vi "angle-statstics-test.vi"(8 "error in (no error)":errorcluster) -> (0 "error out":errorcluster, 3 "All Passed":bool)   [LabVIEW 2019]
uses:
  <vilib>/Analysis/Matrix/Datatypes/RealMatrix.ctl
  <vilib>/Rock Robotics/WPI/ThirdParty/JAS_Junk/TrajLib/MatBuilder_Create.vi
  <vilib>/Rock Robotics/WPI/ThirdParty/JAS_Junk/TrajLib/MathUtil_AngleModulus.vi
  <vilib>/Rock Robotics/WPI/ThirdParty/JAS_Junk/TrajLib/Matrix_ExtractRowVector.vi
  <vilib>/Analysis/baseanly.llb/A x B.vi
  <vilib>/Analysis/baseanly.llb/Real A x B.vi
  <vilib>/Rock Robotics/WPI/ThirdParty/JAS_Junk/TrajLib/Matrix_ElementSum.vi
  <vilib>/Rock Robotics/WPI/ThirdParty/JAS_Junk/TrajLib/MathUtil_InputModulus.vi
  <vilib>/Analysis/Matrix/Numeric/Add/Add.vi
  <vilib>/Analysis/Matrix/Numeric/Add/Add - RM,RM.vi
  <vilib>/Rock Robotics/WPI/ThirdParty/JAS_Junk/TrajLib/Trajectory_Library.lvlib
  <vilib>/Analysis/Matrix/NI_Matrix.lvlib
panel:
  out "Passed 3A":bool
  out "Passed 3":bool
  out "Passed 2A":bool
  out "Passed 2":bool
  out "Passed 1A":bool
  out "Passed 1":bool
  out "Error1":bool
  out "Error 3A":bool
  out "Result 3A":T1
  out "Result 3":T1
  out "Error 2A":bool
  out "Result 2A":T1
  out "Result 2":T1
  out "Error 1A":bool
  out "Result 1A":T1
  out "Result 1":T1
  # "MEAN"
  # "RESIDUAL (MINUS)"
  # "ADD"
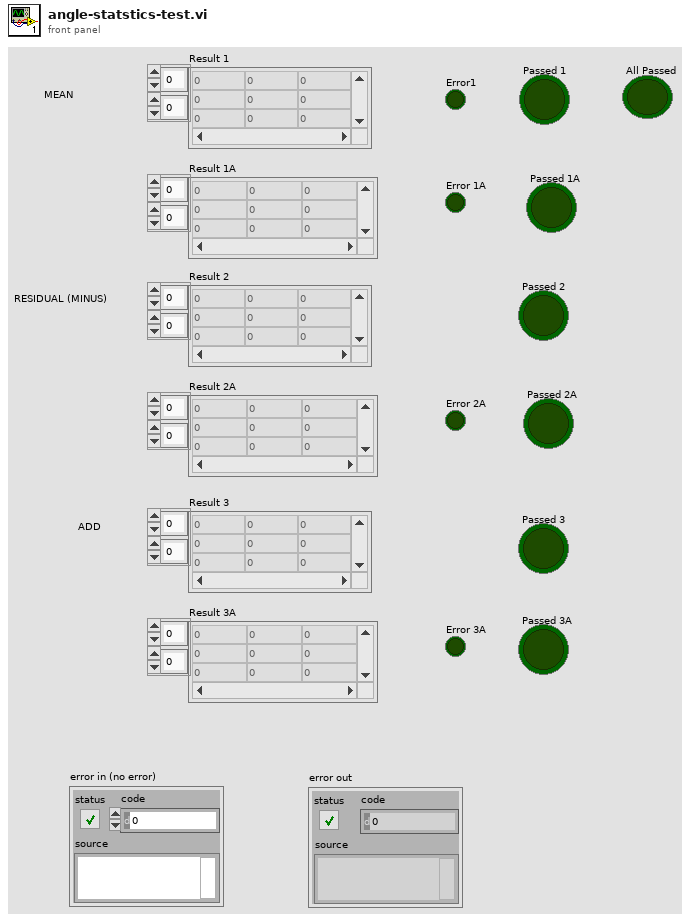
[diagram p1: front panel]
types:
  T1 = typedef "NI_Matrix.lvlib/RealMatrix.ctl" = dbl[][]
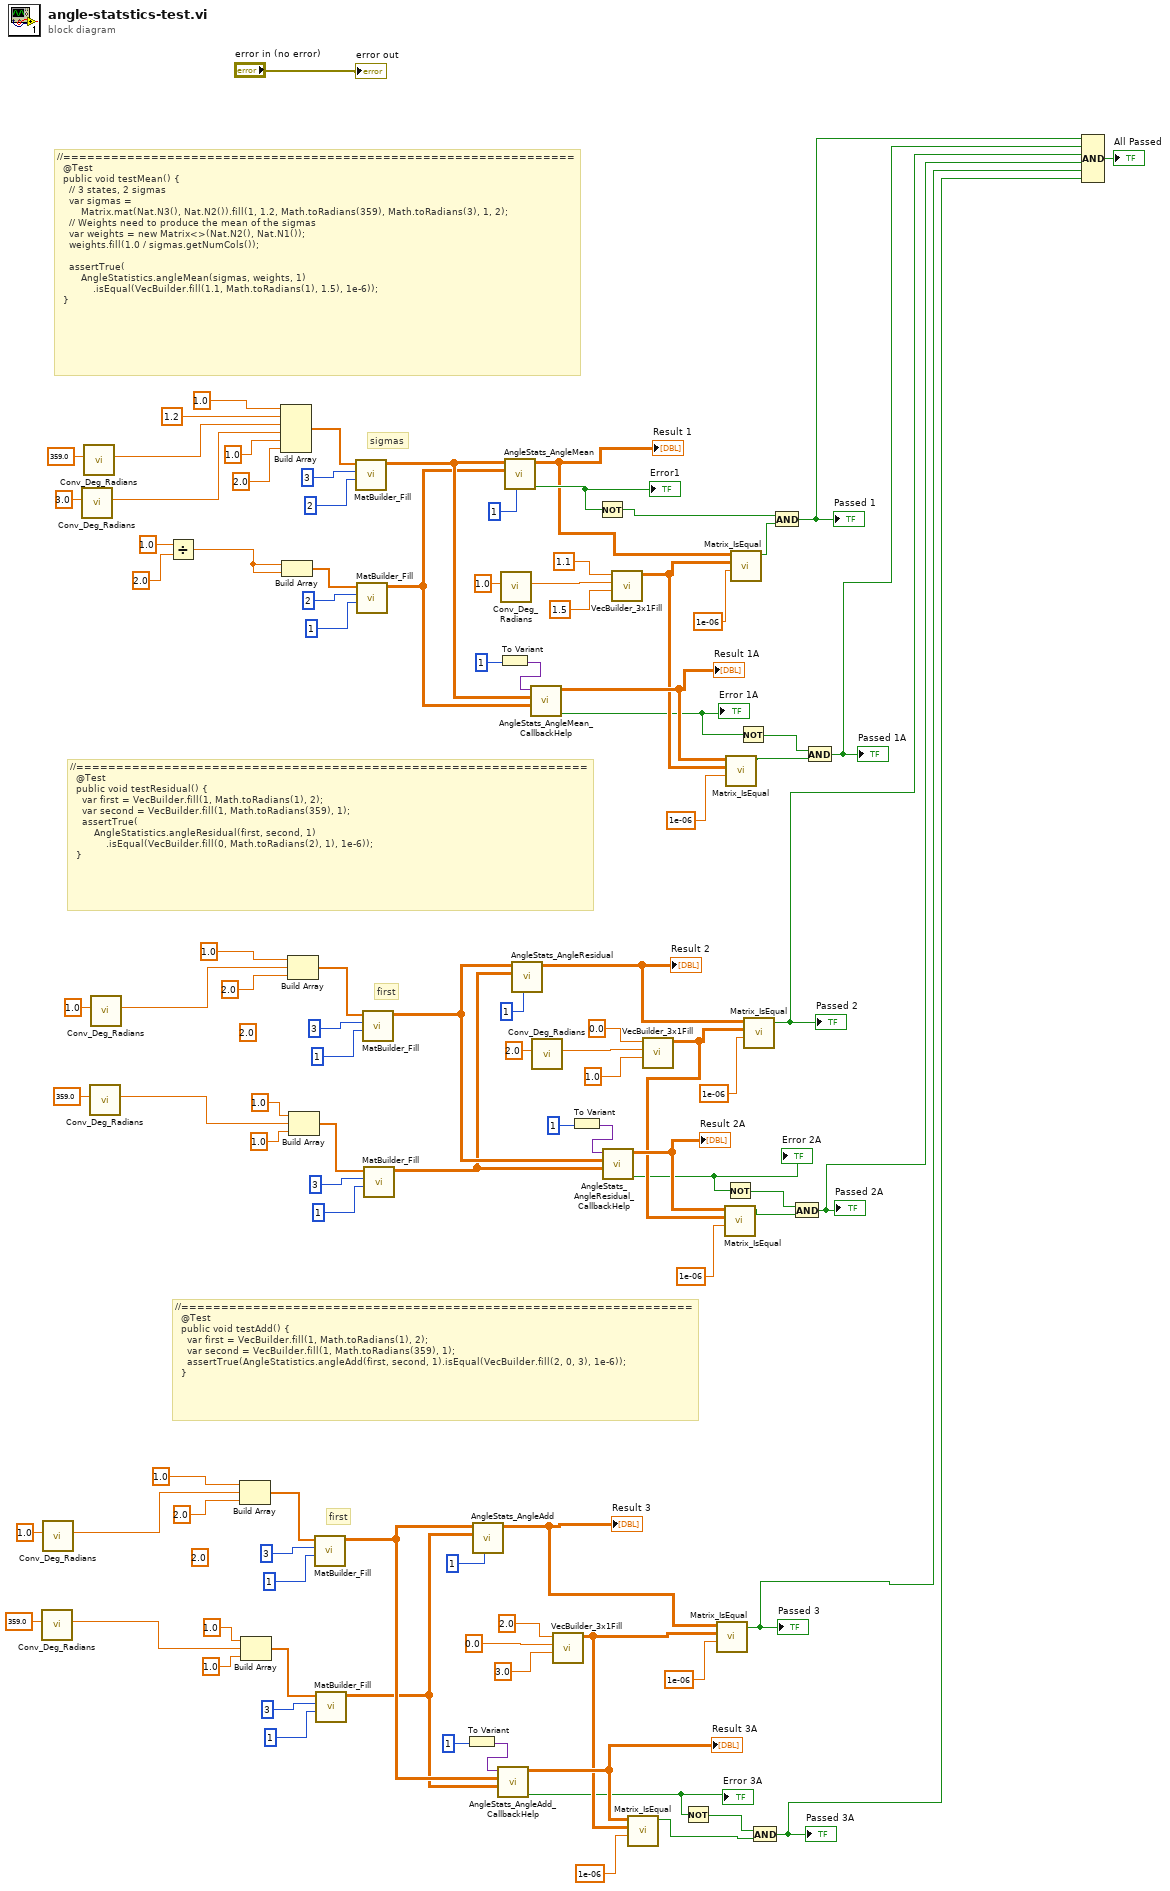
[diagram p0: block diagram]
diagram:
  (unwired) 2.0 ("element")
  (unwired) 2.0 ("element")
  # "first"
  # "//================================================================\n  @Test\n  public void testAdd() {\n    var first = VecBuilder.fill(1, Math.toRadians(1), 2);\n    var second = VecBuilder.fill(1, Math.toRadians(359), 1);\n    assertTrue(AngleStatistics.angleAdd(first, second, 1).isEqual(VecBuilder.fill(2, 0, 3), 1e-6));\n  }"
  # "first"
  # "//================================================================\n  @Test\n  public void testResidual() {\n    var first = VecBuilder.fill(1, Math.toRadians(1), 2);\n    var second = VecBuilder.fill(1, Math.toRadians(359), 1);\n    assertTrue(\n        AngleStatistics.angleResidual(first, second, 1)\n            .isEqual(VecBuilder.fill(0, Math.toRadians(2), 1), 1e-6));\n  }"
  # "sigmas"
  # "//================================================================\n  @Test\n  public void testMean() {\n    // 3 states, 2 sigmas\n    var sigmas =\n        Matrix.mat(Nat.N3(), Nat.N2()).fill(1, 1.2, Math.toRadians(359), Math.toRadians(3), 1, 2);\n    // Weights need to produce the mean of the sigmas\n    var weights = new Matrix<>(Nat.N2(), Nat.N1());\n    weights.fill(1.0 / sigmas.getNumCols());\n\n    assertTrue(\n        AngleStatistics.angleMean(sigmas, weights, 1)\n            .isEqual(VecBuilder.fill(1.1, Math.toRadians(1), 1.5), 1e-6));\n  }"
  n1 = call <vilib>:"Conv_Deg_Radians.vi"("Degress"=359.0) -> ("Radians"=w47:dbl)  [unwired: 10 in]
  n2 = call <vilib>:"Conv_Deg_Radians.vi"("Degress"=1.0) -> ("Radians"=w50:dbl)  [unwired: 10 in]
  n3 = call <vilib>:"Conv_Deg_Radians.vi"("Degress"=3.0) -> ("Radians"=w98:dbl)  [unwired: 10 in]
  n4 = call <vilib>:"Conv_Deg_Radians.vi"("Degress"=359.0) -> ("Radians"=w99:dbl)  [unwired: 10 in]
  n5 = call <vilib>:"Conv_Deg_Radians.vi"("Degress"=359.0) -> ("Radians"=w66:dbl)  [unwired: 10 in]
  n6 = call <vilib>:"Conv_Deg_Radians.vi"("Degress"=1.0) -> ("Radians"=w69:dbl)  [unwired: 10 in]
  n7 = Divide(x=1.0, y=2.0) -> (x/y=w91:dbl)
  n8 = Build Array(1.0 ("element"), w50, 2.0 ("element")) -> (w62:dbl[])
  n9 = Build Array(1.0 ("element"), w47, 1.0 ("element")) -> (w56:dbl[])
  n10 = Build Array(1.0 ("element"), 1.2 ("element"), w99, w98, 1.0 ("element"), 2.0 ("element")) -> (w104:dbl[])
  n11 = Build Array(w91, w91) -> (w90:dbl[])
  n12 = Build Array(1.0 ("element"), w69, 2.0 ("element")) -> (w81:dbl[])
  n13 = Build Array(1.0 ("element"), w66, 1.0 ("element")) -> (w75:dbl[])
  n14 = call <vilib>:"MatBuilder_Fill.vi"("Columns"=1, "Rows"=3, "Value List"=w62) -> ("output matrix"=w54:T1)  [unwired: 8 in]
  n15 = call <vilib>:"MatBuilder_Fill.vi"("Columns"=1, "Rows"=3, "Value List"=w56) -> ("output matrix"=w53:T1)  [unwired: 8 in]
  n16 = call <vilib>:"MatBuilder_Fill.vi"("Columns"=2, "Rows"=3, "Value List"=w104) -> ("output matrix"=w88:T1)  [unwired: 8 in]
  n17 = call <vilib>:"MatBuilder_Fill.vi"("Columns"=1, "Rows"=2, "Value List"=w90) -> ("output matrix"=w87:T1)  [unwired: 8 in]
  n18 = call <vilib>:"MatBuilder_Fill.vi"("Columns"=1, "Rows"=3, "Value List"=w81) -> ("output matrix"=w73:T1)  [unwired: 8 in]
  n19 = call <vilib>:"MatBuilder_Fill.vi"("Columns"=1, "Rows"=3, "Value List"=w75) -> ("output matrix"=w72:T1)  [unwired: 8 in]
  n20 = To Variant(anything=1) -> (Variant=w51:variant)
  n21 = call <vilib>:"AngleStats_AngleAdd.vi"("Row"=1, "B"=w53, "A"=w54) -> ("Result"=w16:T1)  [unwired: 8 in]
  "Result 3" <- w16
  n22 = call <vilib>:"AngleStats_AngleAdd_CallbackHelp.vi"("B"=w53, "A"=w54, "ExtraPassedData"=w51) -> ("Error"=w9:bool, "Result"=w13:T1)  [unwired: 7 in]
  "Result 3A" <- w13
  "Error 3A" <- w9
  n23 = To Variant(anything=1) -> (Variant=w84:variant)
  n24 = call <vilib>:"Conv_Deg_Radians.vi"("Degress"=1.0) -> ("Radians"=w44:dbl)  [unwired: 10 in]
  n25 = call <vilib>:"AngleStats_AngleMean.vi"("Row"=1, "Wm"=w87, "Sigmas"=w88) -> ("Error"=w41:bool, "Result"=w39:T1)  [unwired: 7 in]
  "Result 1" <- w39
  "Error1" <- w41
  n26 = call <vilib>:"AngleStats_AngleResidual.vi"("Row"=1, "B"=w72, "A"=w73) -> ("Result"=w26:T1)  [unwired: 8 in]
  "Result 2" <- w26
  n27 = call <vilib>:"AngleStats_AngleMean_CallbackHelp.vi"("B"=w87, "A"=w88, "ExtraPassedData"=w84) -> ("Error"=w34:bool, "Result"=w36:T1)  [unwired: 7 in]
  "Result 1A" <- w36
  "Error 1A" <- w34
  n28 = call <vilib>:"Conv_Deg_Radians.vi"("Degress"=2.0) -> ("Radians"=w29:dbl)  [unwired: 10 in]
  n29 = call <vilib>:"VecBuilder_3x1Fill.vi"("R2"=3.0, "R1"=0.0 ("Degress"), "R0"=2.0) -> ("output matrix"=w12:T1)  [unwired: 8 in]
  n30 = To Variant(anything=1) -> (Variant=w70:variant)
  n31 = Not(x=w41) -> (.not. x?=w40:bool)
  n32 = call <vilib>:"AngleStats_AngleResidual_CallbackHelp.vi"("B"=w72, "A"=w73, "ExtraPassedData"=w70) -> ("Error"=w21:bool, "Result"=w24:T1)  [unwired: 7 in]
  "Result 2A" <- w24
  "Error 2A" <- w21
  n33 = call <vilib>:"VecBuilder_3x1Fill.vi"("R2"=1.5, "R1"=w44, "R0"=1.1) -> ("output matrix"=w35:T1)  [unwired: 8 in]
  n34 = call <vilib>:"Matrix_IsEqual.vi"("Tolerance"=1e-06, "other"=w12, "input matrix"=w13) -> ("Equal"=w10:bool)  [unwired: 8 in]
  n35 = call <vilib>:"VecBuilder_3x1Fill.vi"("R2"=1.0, "R1"=w29, "R0"=0.0) -> ("output matrix"=w23:T1)  [unwired: 8 in]
  n36 = Not(x=w9) -> (.not. x?=w11:bool)
  n37 = call <vilib>:"Matrix_IsEqual.vi"("Tolerance"=1e-06, "other"=w12, "input matrix"=w16) -> ("Equal"=w4:bool)  [unwired: 8 in]
  "Passed 3" <- w4
  n38 = Not(x=w21) -> (.not. x?=w22:bool)
  n39 = call <vilib>:"Matrix_IsEqual.vi"("Tolerance"=1e-06, "other"=w23, "input matrix"=w24) -> ("Equal"=w20:bool)  [unwired: 8 in]
  n40 = call <vilib>:"Matrix_IsEqual.vi"("Tolerance"=1e-06, "other"=w35, "input matrix"=w36) -> ("Equal"=w33:bool)  [unwired: 8 in]
  n41 = call <vilib>:"Matrix_IsEqual.vi"("Tolerance"=1e-06, "other"=w35, "input matrix"=w39) -> ("Equal"=w38:bool)  [unwired: 8 in]
  n42 = Not(x=w34) -> (.not. x?=w32:bool)
  n43 = call <vilib>:"Matrix_IsEqual.vi"("Tolerance"=1e-06, "other"=w23, "input matrix"=w26) -> ("Equal"=w6:bool)  [unwired: 8 in]
  "Passed 2" <- w6
  n44 = And(x=w11, y=w10) -> (x .and. y?=w3:bool)
  "Passed 3A" <- w3
  n45 = And(x=w40, y=w38) -> (x .and. y?=w8:bool)
  "Passed 1" <- w8
  n46 = And(x=w22, y=w20) -> (x .and. y?=w5:bool)
  "Passed 2A" <- w5
  n47 = And(x=w32, y=w33) -> (x .and. y?=w7:bool)
  "Passed 1A" <- w7
  n48 = Compound Arithmetic op=AND(w8, w7, w6, w5, w4, w3) -> (→"All Passed":bool)
  "error out" <- "error in (no error)"
